vi "MeasureImageSharpness.vi"(8 "error in (no error)":errorcluster, 10 "Method":T2(ring), 11 "Image In":T1) -> (0 "error out":errorcluster, 1 "Sharpness Uncertainty":dbl, 2 "Sharpness":dbl, 3 "Image Out":T1)   [LabVIEW 2016]
uses:
  <vilib>/vision/Image Controls.llb/IMAQ Image.ctl
  <vilib>/vision/NI_Vision_Development_Module.lvlib
panel:
  in  "Tab Control":enum32{"Processing", "Test settings"}(tab)
  in  "Testing?":bool
  in  "Test Image Path":path
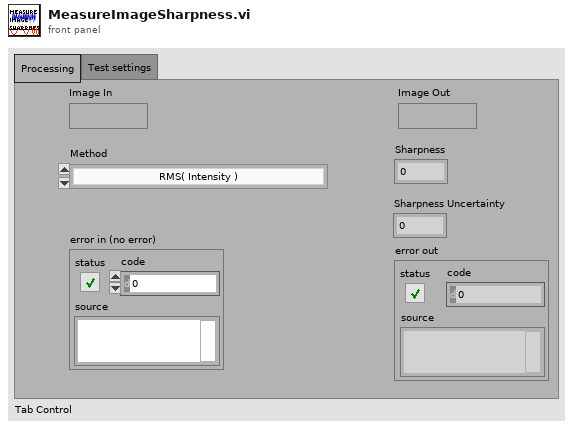
[diagram p1: front panel]
types:
  T1 = typedef "IMAQ Image.ctl" = refnum<image>
  T2 = enum16{"RMS( Intensity )", "Mean( Laplacian Convolution )"}
  T3 = cluster{"histogram":u32[], "Minimal Value":sgl, "Maximal Value":sgl, "Starting Value":sgl, "Interval Width":sgl, "Mean Value":sgl, "Standard  Variation":sgl, "Area (pixels)":i32}
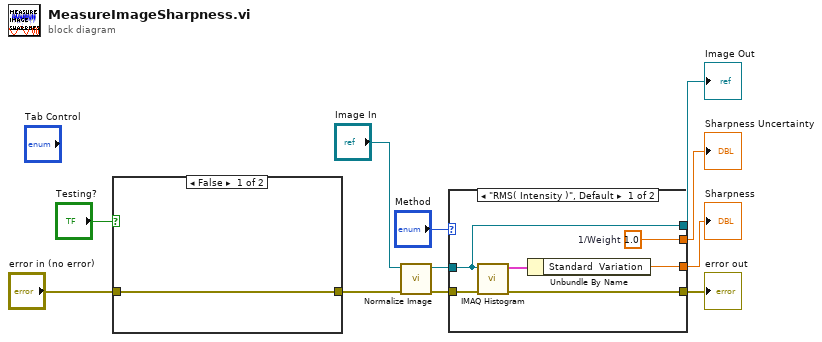
[diagram p0: block diagram]
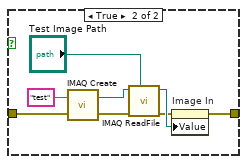
[diagram p2: hidden frame]
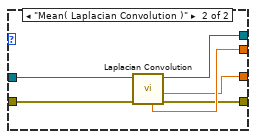
[diagram p3: hidden frame]
diagram:
  n1 = case shown="False" "Testing?" {
    tunnel: [w12 w16] -> w4
    tunnel: "error in (no error)" -> [w12 w13]
    frame False {
    }
    frame True {
      n2 = call "IMAQ Create"("Image Name"="test", "error in (no error)"=w13) -> ("New Image"=w20:T1, "error out"=w14:errorcluster)  [unwired: 3 in]
      n3 = call "IMAQ ReadFile"("File Path"="Test Image Path", "error in (no error)"=w14, "Image"=w20) -> ("error out"=w15:errorcluster, "Image Out"=w18:T1)  [unwired: 4 in, 3 out]
      n4 = property on="Image In" class="IMAQImage (strict)"(error in=w15, "Value"=w18) -> (error out=w16:errorcluster)  [unwired: 1 in, 1 out]
    }
  }
  n5 = call "Normalize Image.vi"("error in (no error)"=w4, "Image In"="Image In") -> ("error out"=w8:errorcluster, "Image Out"=w9:T1)  [unwired: 8 in]
  n6 = case shown="\"RMS( Intensity )\", Default" "Method" {
    tunnel: w9 -> [w24 w32]
    tunnel: w8 -> [w26 w31]
    tunnel: [w24 w30] -> w7
    tunnel: [w22 w29] -> w6
    tunnel: [w21 w28] -> w5
    tunnel: [w23 w27] -> w1
    frame "RMS( Intensity )", Default {
      w22 = sgl 1.0  # 1/Weight
      n7 = call "IMAQ Histogram"("error in (no error)"=w26, "Image"=w24) -> ("error out"=w23:errorcluster, "Histogram Report"=w25:T3)  [unwired: 8 in]
      n8 = Unbundle By Name(w25) -> ("Standard  Variation"=w21:sgl)
    }
    frame "Mean( Laplacian Convolution )" {
      n9 = call "Laplacian Convolution.vi"("error in (no error)"=w31, "Refnum in"=w32) -> ("error out"=w27:errorcluster, "Mean Value"=w28:sgl, "Refnum out"=w30:T1, "Standard  Variation"=w29:sgl)  [unwired: 4 in, 2 out]
    }
  }
  "Image Out" <- w7
  "error out" <- w1
  "Sharpness" <- w5
  "Sharpness Uncertainty" <- w6
